vi "save_fp.vi"(7 "Image Type":enum16{"JPEG", "PNG", "BMP"}(ring), 8 "error in":errorcluster, 10 "Image Path":path) -> (0 "error out":errorcluster)   [LabVIEW 2014]
uses:
  <vilib>/Utility/sysdir.llb/System Directory Type.ctl
  type definitions/control camera properties.ctl
panel:
  in  "input cluster 2":T1={"Packet Size"=1500, "Pixel Format"=17825797, "Gain in dB"=1.0, "Exposure Time in µs"=1500, "Stream Bytes per Second"=50000017} caption="Control Camera Properties" {"Stream Bytes per Second" min=1000000 max=124000000 step=100000 format="%.1p"; "Exposure Time in µs" min=21 max=153391689 format="%#.0f"; "Gain in dB" min=0.0 max=26.0 format="%#_2g"; "Pixel Format" items=["Mono 12 Packed"=17563654, "Mono 12"=17825797]}
  in  "input cluster":T2
  out "Image Pixels (U16)":u16[][](graph)
  in  "Image Pixels (U16) 3":u16[][](graph)
  in  "file path":path
  in  "base path":path
  in  "Image Pixels (U16) 2":u16[][](graph)
  # "Bytes"
  # "Trigger"
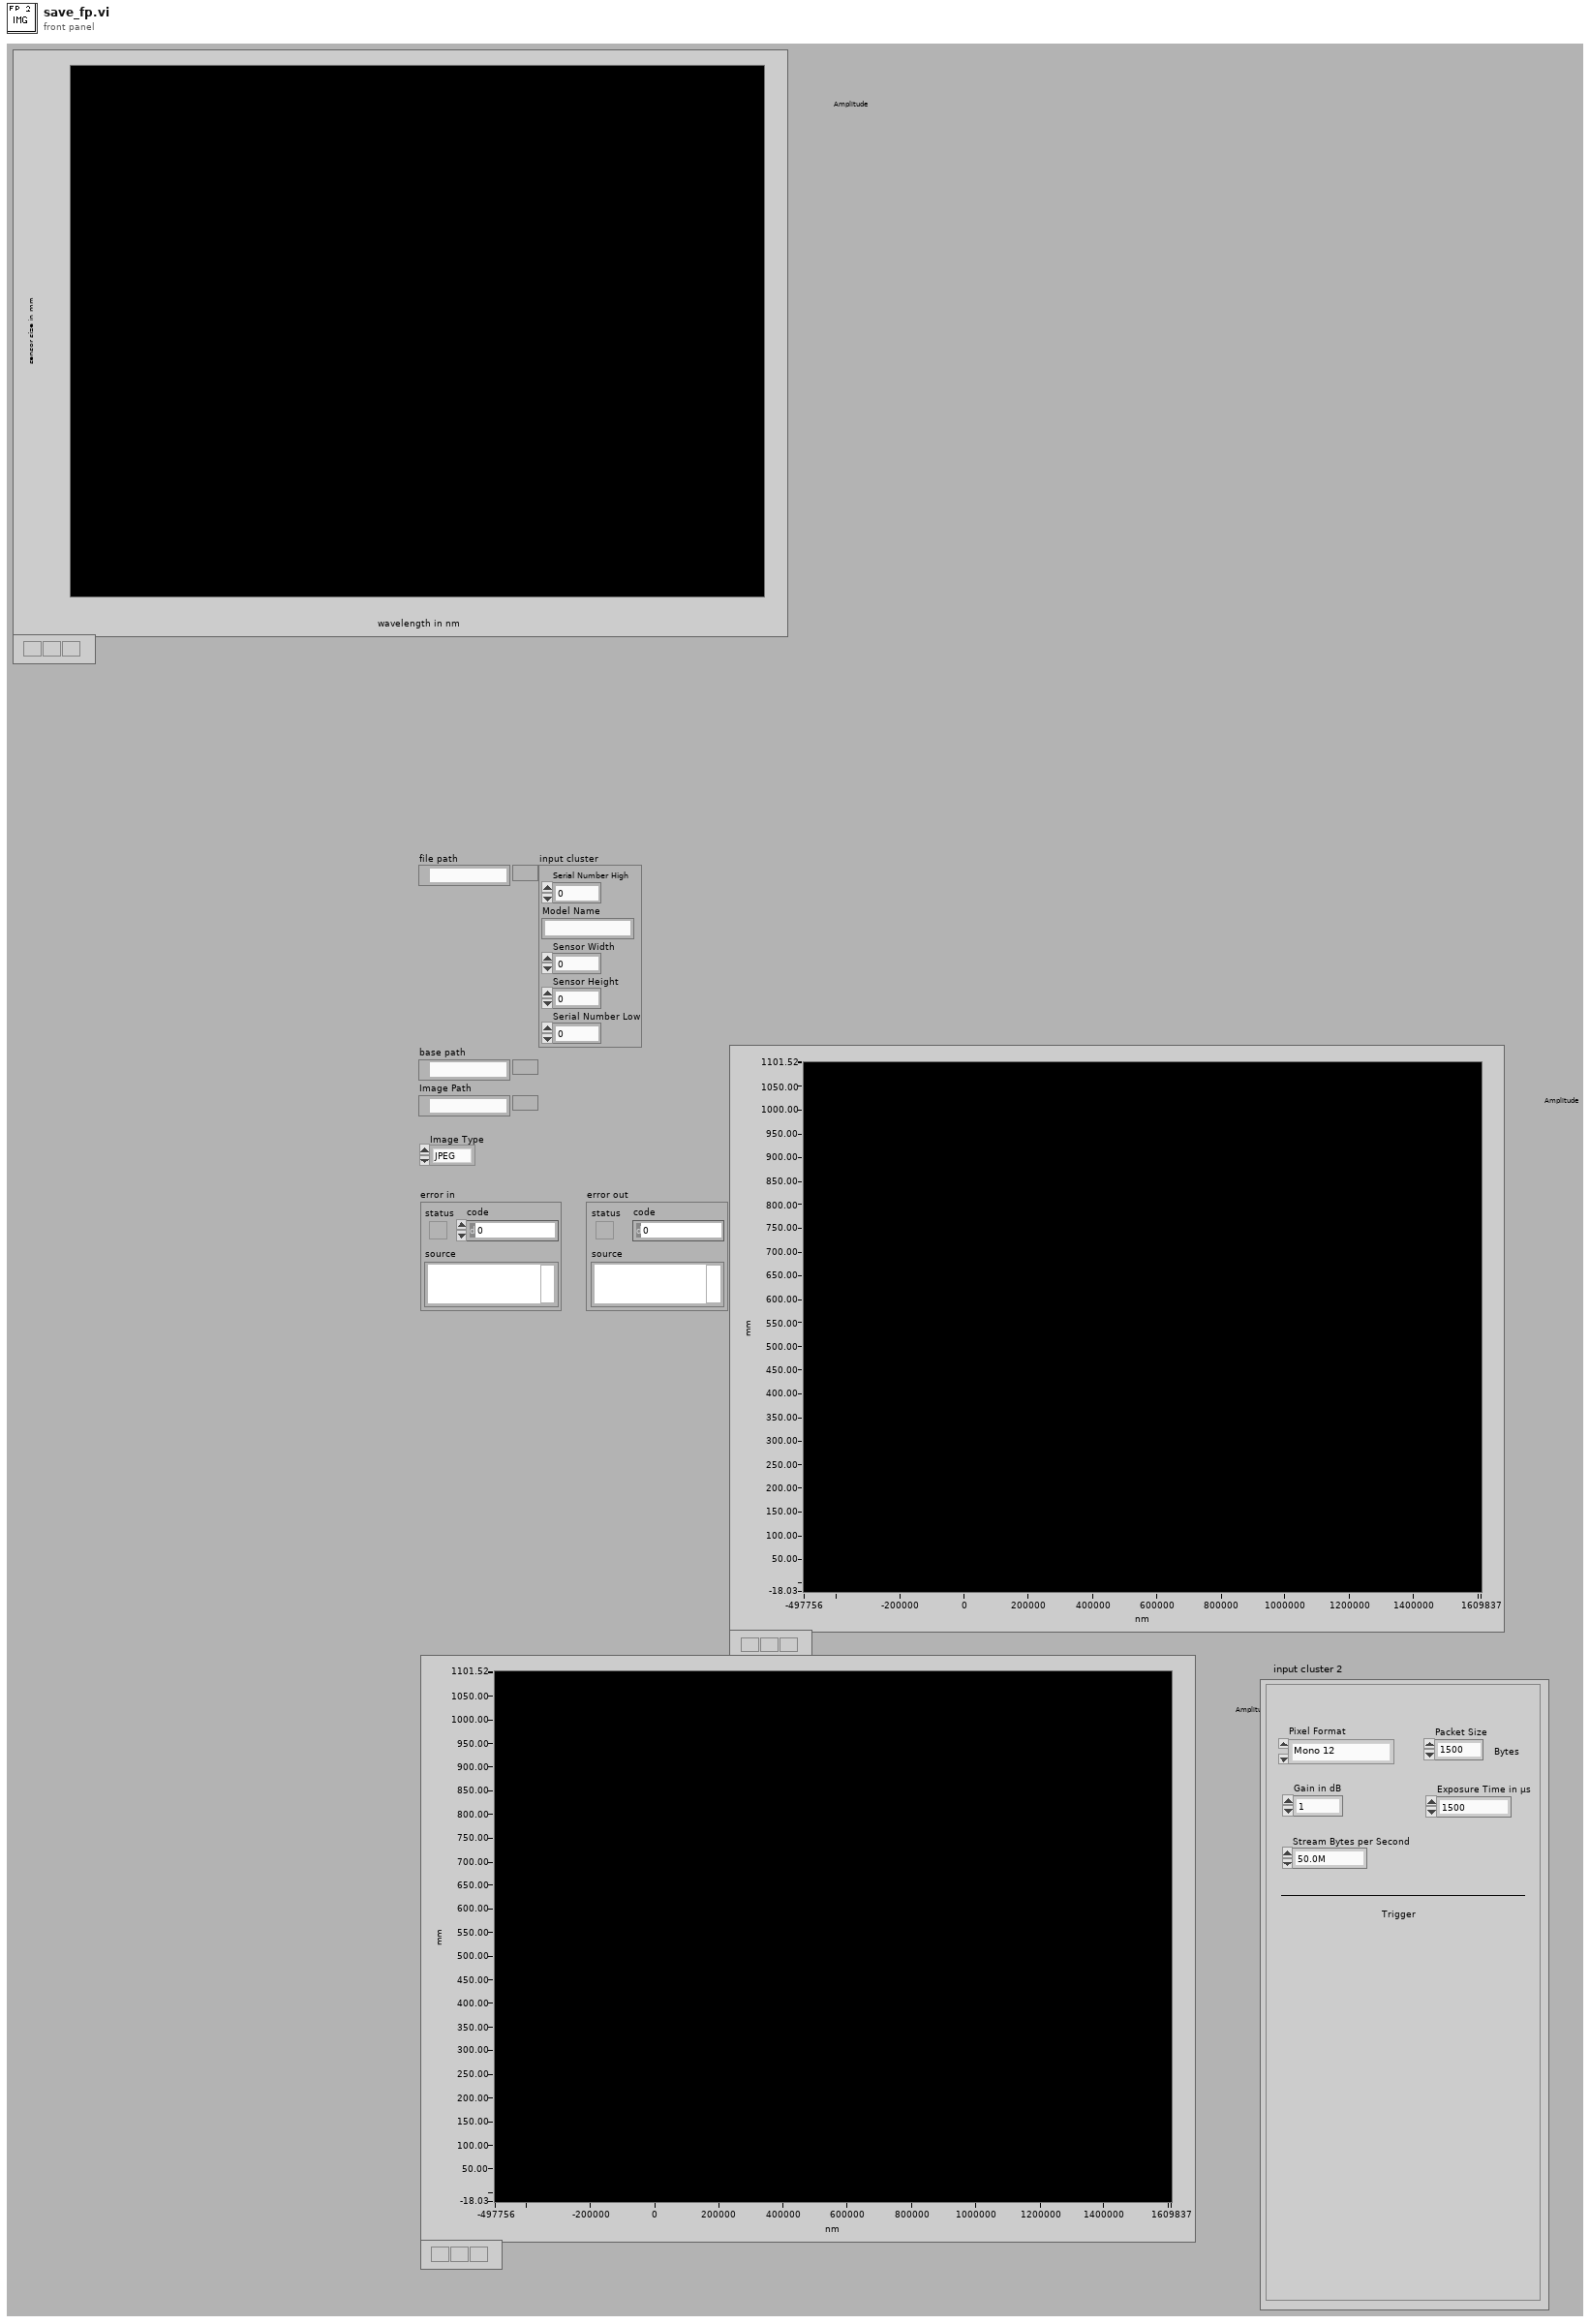
[diagram p1: front panel]
types:
  T1 = typedef "control camera properties.ctl" = cluster{"Packet Size":u32, "Pixel Format":u32, "Gain in dB":dbl, "Exposure Time in µs":u32, "Stream Bytes per Second":u32}
  T2 = cluster{"Serial Number High":u32, "Model Name":string, "Sensor Width":u32, "Sensor Height":u32, "Serial Number Low":u32}
  T3 = enum16{"open", "open or create", "create or replace", "create", "open (read-only)"}
  T4 = typedef "System Directory Type.ctl" = i32
  T5 = enum16{"open", "replace", "create", "open or create", "replace or create", "replace or create with confirmation"}
  T6 = typedef "imagedata.ctl" = cluster{"image type":i32, "image depth":i32, "image":u8[], "mask":u8[], "colors":u32[], "Rectangle":cluster{"left":i16, "top":i16, "right":i16, "bottom":i16}}
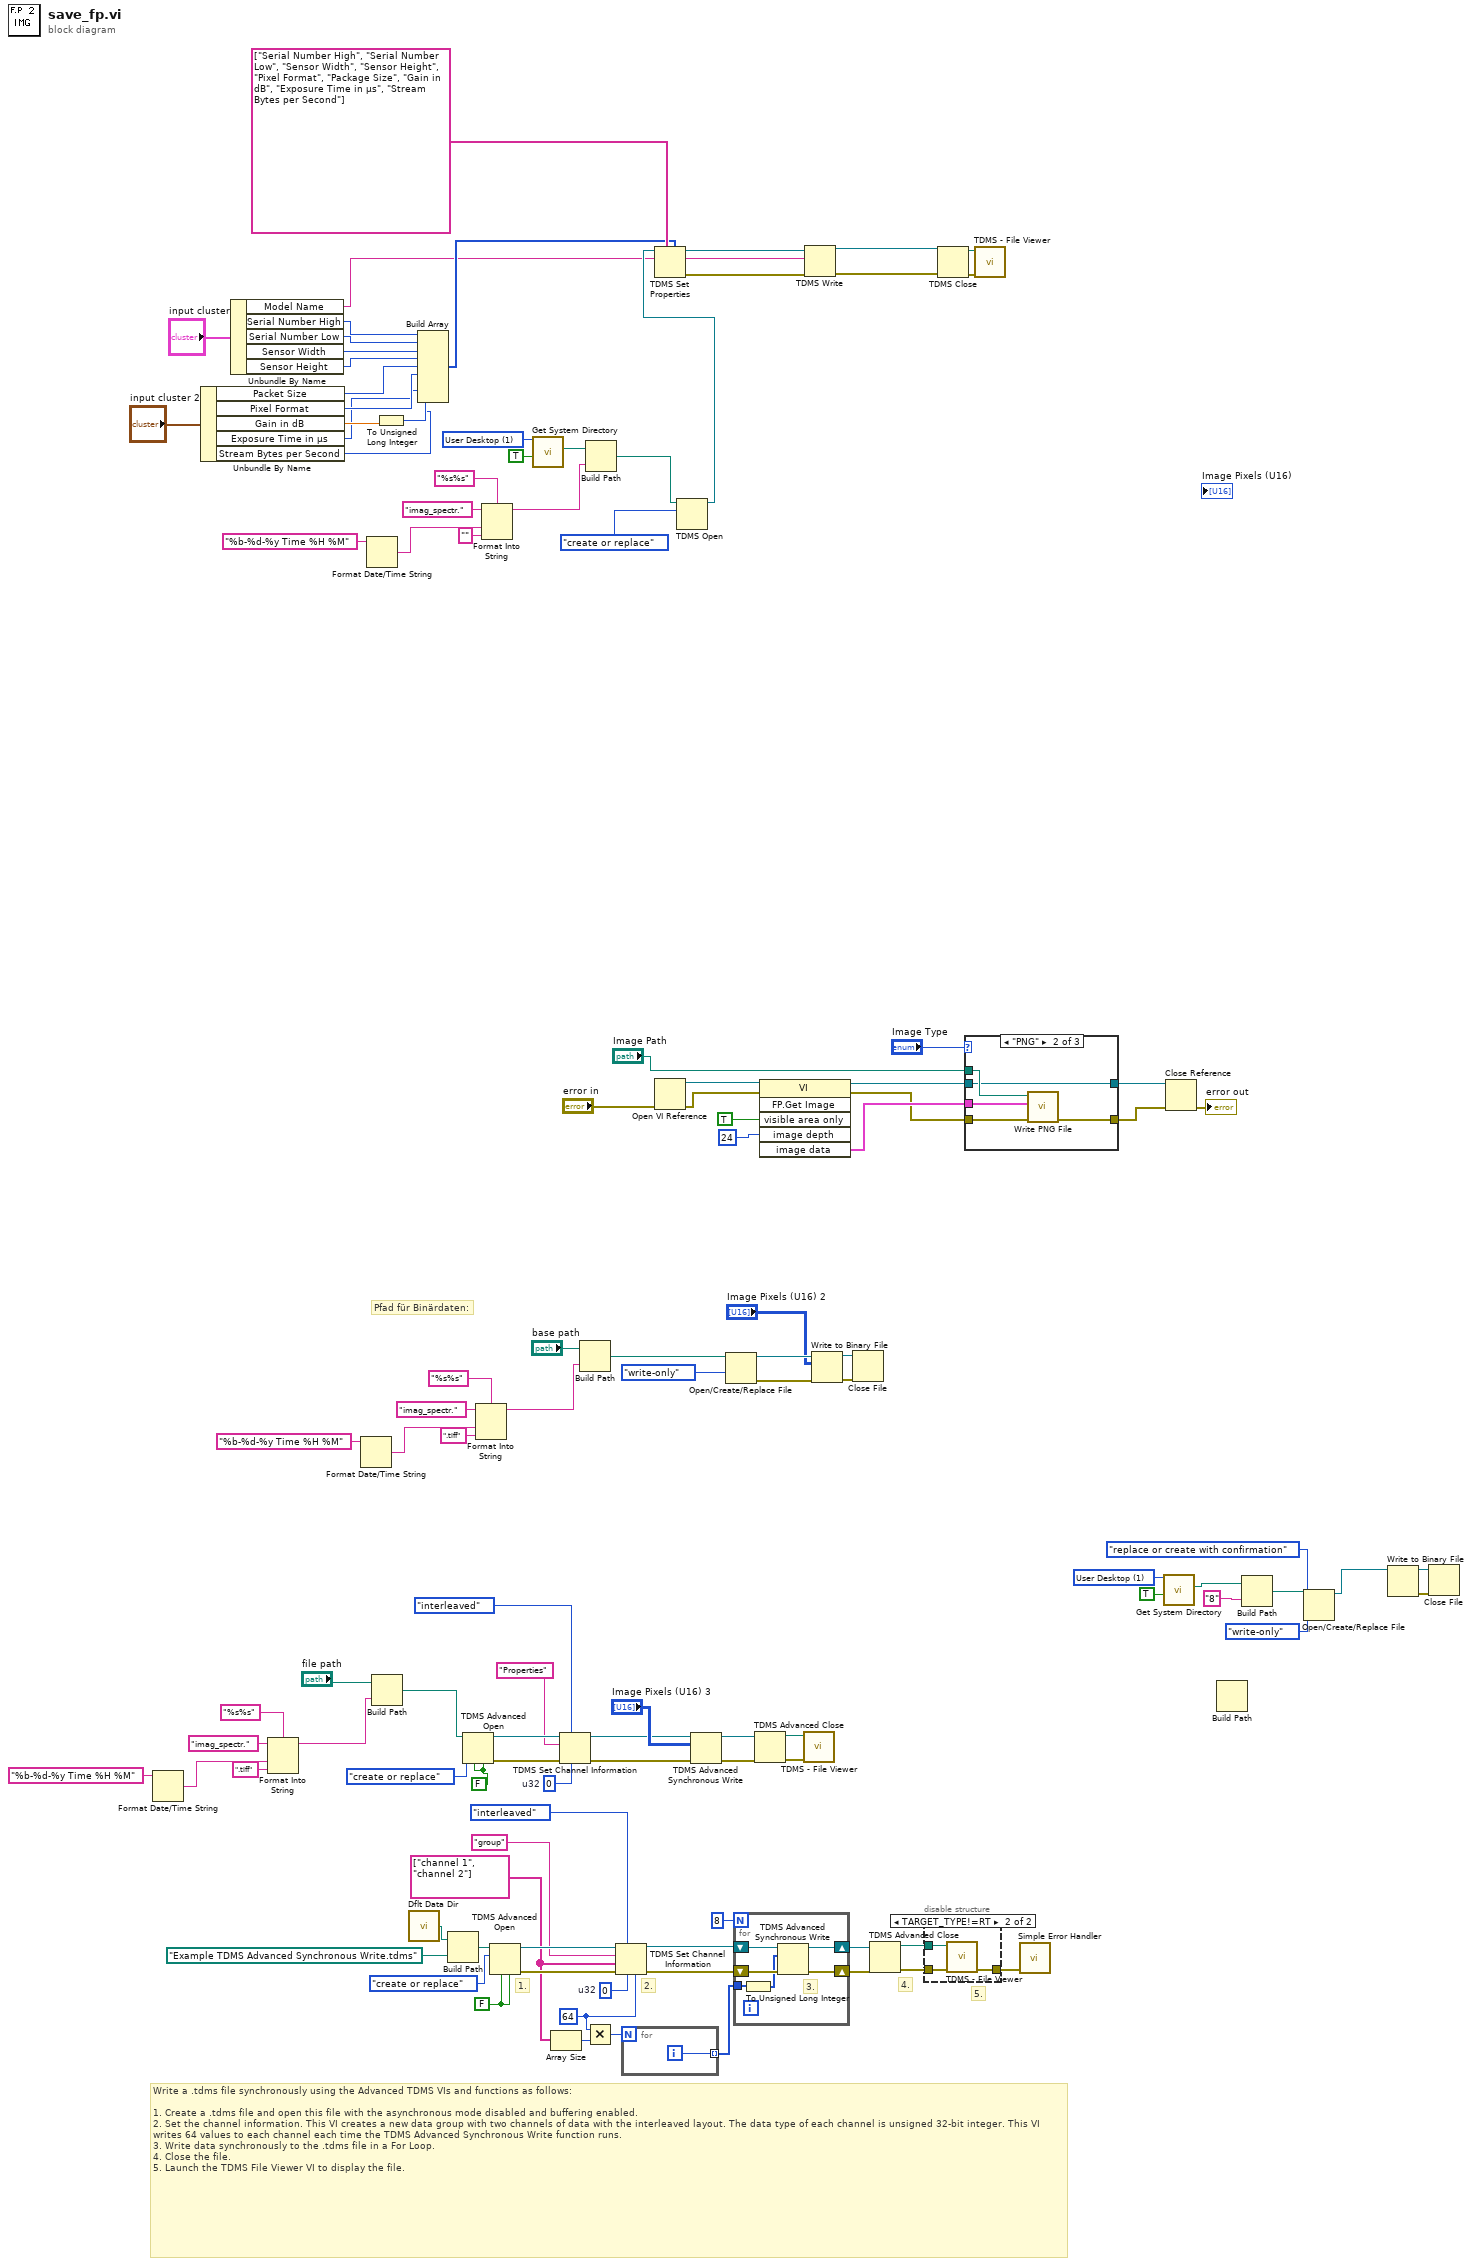
[diagram p0: block diagram]
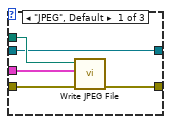
[diagram p3: hidden frame]
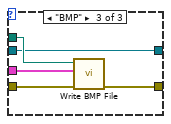
[diagram p4: hidden frame]
diagram:
  w27 = T4 1 items=["User Home"=0, "User Desktop"=1, "User Documents"=2, "User Application Data"=3, "User Preferences"=4, "User Temporary"=5, "Public Documents"=6, "Public Application Data"=7, "Public Preferences"=8, "Public Cache"=13, "System Core Libraries"=9, "System Installed Libraries"=10, "Application Files"=11, "Boot Volume Root"=12] ("system directory type")
  w38 = T4 1 items=["User Home"=0, "User Desktop"=1, "User Documents"=2, "User Application Data"=3, "User Preferences"=4, "User Temporary"=5, "Public Documents"=6, "Public Application Data"=7, "Public Preferences"=8, "Public Cache"=13, "System Core Libraries"=9, "System Installed Libraries"=10, "Application Files"=11, "Boot Volume Root"=12] ("system directory type")
  w56 = u32 0  # u32
  w57 = FALSE
  w76 = FALSE ("enable asynchronous? (T)")
  w66 = u32 64 ("samples per channel")
  w77 = u32 0  # u32
  w67 = string[] ["channel 1", "channel 2"] ("channel name(s)")
  # "Write a .tdms file synchronously using the Advanced TDMS VIs and functions as follows:\n\n1. Create a .tdms file and open this file with the asynchronous mode disabled and buffering enabled.\n2. Set the channel information. This VI creates a new data group with two channels of data with the interleaved layout. The data type of each channel is unsigned 32-bit integer. This VI writes 64 values to each channel each time the TDMS Advanced Synchronous Write function runs.\n3. Write data synchronously to the .tdms file in a For Loop.\n4. Close the file.\n5. Launch the TDMS File Viewer VI to display the file."
  # "5."
  # "1."
  # "4."
  # "2."
  # "Pfad für Binärdaten:"
  n1 = Format Date/Time String(time format string (%c)="%b-%d-%y Time %H %M") -> (date/time string=w60:string)  [unwired: 2 in]
  n2 = Unbundle By Name("input cluster 2") -> ("Packet Size"=w11:u32, "Pixel Format"=w10:u32, "Gain in dB"=w9:dbl, "Exposure Time in µs"=w7:u32, "Stream Bytes per Second"=w6:u32)
  n3 = Unbundle By Name("input cluster") -> ("Model Name"=w4:string, "Serial Number High"=w15:u32, "Serial Number Low"=w14:u32, "Sensor Width"=w13:u32, "Sensor Height"=w12:u32)
  n4 = Format Into String(format string="%s%s", initial string="imag_spectr.", w60, ".tiff" ("input 2")) -> (resulting string=w65:string)  [unwired: 1 in, 1 out]
  n5 = Format Date/Time String(time format string (%c)="%b-%d-%y Time %H %M") -> (date/time string=w103:string)  [unwired: 2 in]
  n6 = Format Date/Time String(time format string (%c)="%b-%d-%y Time %H %M") -> (date/time string=w21:string)  [unwired: 2 in]
  n7 = Build Path(base path="file path", name or relative path=w65) -> (appended path=w58:path)
  n8 = To Unsigned Long Integer(number=w9) -> (unsigned 32bit integer=w8:u32)
  n9 = call <vilib>:"Dflt Data Dir.vi"() -> ("App:Default Data Directory"=w84:path)
  n10 = Build Array(w15, w14, w13, w12, w11, w10, w8, w7, w6) -> (w5:u32[])
  n11 = Build Path(base path=w84, name or relative path=path "Example TDMS Advanced Synchronous Write.tdms") -> (appended path=w88:path)
  n12 = TDMS Advanced Open(4:w57, 6:w57, 10:T3."create or replace" ("operation (0:open)"), 11:w58) -> (0:w55:errorcluster, 3:w54:refnum<k34>)  [unwired: 1 in, 1 out]
  n13 = Format Into String(format string="%s%s", initial string="imag_spectr.", w103, ".tiff" ("input 2")) -> (resulting string=w89:string)  [unwired: 1 in, 1 out]
  n14 = Format Into String(format string="%s%s", initial string="imag_spectr.", w21, "" ("input 2")) -> (resulting string=w25:string)  [unwired: 1 in, 1 out]
  n15 = TDMS Advanced Open(4:w76, 6:w76, 10:T3."create or replace" ("operation (0:open)"), 11:w88) -> (0:w86:errorcluster, 3:w85:refnum<k34>)  [unwired: 1 in, 1 out]
  n16 = call <vilib>:"Get System Directory.vi"("create directory if not found? (F)"=TRUE, "system directory type"=w27) -> ("system directory"=w20:path)  [unwired: 9 in]
  n17 = Array Size(array=w67) -> (size(s)=w69:i32)
  n18 = TDMS Set Channel Information(6:w56, 7:enum16{"non-interleaved", "interleaved"}."interleaved" ("data layout (0:non-interleaved)"), 8:w55, 10:"Properties" ("group name (Untitled)"), 11:w54) -> (0:w49:errorcluster, 3:w50:refnum<k34>)  [unwired: 2 in]
  n19 = Build Path(base path="base path", name or relative path=w89) -> (appended path=w96:path)
  n20 = Multiply(x=w66, y=w69) -> (x*y=w68:u32)
  n21 = Build Path(base path=w20, name or relative path=w25) -> (appended path=w2:path)
  n22 = TDMS Set Channel Information(4:w66, 6:w77, 7:enum16{"non-interleaved", "interleaved"}."interleaved" ("data layout (0:non-interleaved)"), 8:w86, 9:w67, 10:"group" ("group name (Untitled)"), 11:w85) -> (0:w75:errorcluster, 3:w74:refnum<k34>)
  n23 = for {
    N: w68 -> [_]
    tunnel: [w117] -> w80 mode=indexing
    i -> [w117]
  }
  n24 = Open VI Reference(error in (no error)="error in") -> (vi reference=w114:refnum<vi>, error out=w113:errorcluster)  [unwired: 2 in, 3 out]
  n25 = TDMS Open(10:T3."create or replace" ("operation (0:open)"), 11:w2) -> (3:w18:refnum<k34>)  [unwired: 5 in, 1 out]
  n26 = TDMS Set Properties(5:w5, 7:string[] ["Serial Number High", "Serial Number Low", "Sensor Width", "Sensor Height", "Pixel Format", "Package Size", "Gain in dB", "Exposure Time in µs", "Stream Bytes per Second"] ("property names"), 10:w4, 11:w18) -> (0:w17:errorcluster, 2:w3:string, 3:w16:refnum<k34>)  [unwired: 2 in, 1 out]
  n27 = TDMS Advanced Synchronous Write(8:w49, 10:"Image Pixels (U16) 3", 11:w50) -> (0:w47:errorcluster, 3:w48:refnum<k34>)
  n28 = Open/Create/Replace File(file path (use dialog)=w96, access (0:read/write)=enum16{"read/write", "read-only", "write-only"}."write-only") -> (refnum out=w95:refnum<file>, error out=w92:errorcluster)  [unwired: 4 in, 1 out]
  n29 = for {
    N: 8 -> [_]
    shift-right: [w120] -> w78
    shift-left: w74 -> [w122]
    shift-right: [w121] -> w79
    shift-left: w75 -> [w123]
    tunnel: w80 -> [w119]
    # "3."
    n30 = To Unsigned Long Integer(number=w119) -> (unsigned 32bit integer=w118:u32[])
    n31 = TDMS Advanced Synchronous Write(8:w123, 10:w118, 11:w122) -> (0:w121:errorcluster, 3:w120:refnum<k34>)
  }
  n32 = TDMS Advanced Close(8:w47, 11:w48) -> (0:w46:errorcluster, 3:w45:path)  [unwired: 2 in]
  n33 = invoke class="VI" method="FP.Get Image"(reference=w114, error in=w113, "visible area only"=TRUE ("Visible Area Only"), "image depth"=24 ("Image Depth")) -> (reference out=w107:refnum<vi>, error out=w110:errorcluster, "image data"=w111:T6)  [unwired: 2 in, 3 out]
  n34 = call <vilib>:"TDMS - File Viewer.vi"("error in (no error)"=w46, "file path"=w45) -> ()  [unwired: 6 out]
  n35 = TDMS Write(0:w16, 5:w3, 11:w17) -> (4:w30:refnum<k34>, 15:w31:errorcluster)  [unwired: 3 in, 2 out]
  n36 = Write to Binary File(file (use dialog)=w95, data="Image Pixels (U16) 2", error in=w92) -> (refnum out=w94:refnum<file>, error out=w97:errorcluster)  [unwired: 3 in, 1 out]
  n37 = Close File(refnum=w94, error in=w97) -> ()  [unwired: 2 out]
  n38 = TDMS Advanced Close(8:w79, 11:w78) -> (0:w71:errorcluster, 3:w72:path)  [unwired: 2 in]
  n39 = disable-structure shown="TARGET_TYPE!=RT" {
    disable-tunnel: w71 -> [w124 w127]
    disable-tunnel: w72 -> [_ w126]
    disable-tunnel: [w124 w125] -> w70
    frame condition #0 {
    }
    frame condition #1 (active) {
      n40 = call <vilib>:"TDMS - File Viewer.vi"("error in (no error)"=w127, "file path"=w126) -> ("error out"=w125:errorcluster)  [unwired: 5 out]
    }
  }
  n41 = TDMS Close(8:w31, 11:w30) -> (0:w32:errorcluster, 3:w29:path)
  n42 = case shown="\"PNG\"" "Image Type" {
    tunnel: w111 -> [w131 w137 w141]
    tunnel: w110 -> [w132 w136 w142]
    tunnel: "Image Path" -> [w130 w135 w140]
    tunnel: [w128 w134 w139] -> w108
    tunnel: w107 -> [w129 w133 w138]
    tunnel: [w129 w133 w138] -> w106
    frame "JPEG", Default {
      n43 = call <vilib>:"Write JPEG File.vi"("error in (no error)"=w132, "image data"=w131, "path to JPEG file"=w130) -> ("error out"=w128:errorcluster)  [unwired: 8 out]
    }
    frame "PNG" {
      n44 = call <vilib>:"Write PNG File.vi"("error in (no error)"=w136, "image data"=w137, "path to PNG file"=w135) -> ("error out"=w134:errorcluster)  [unwired: 8 out]
    }
    frame "BMP" {
      n45 = call <vilib>:"Write BMP File.vi"("error in (no error)"=w142, "image data"=w141, "path to BMP file"=w140) -> ("error out"=w139:errorcluster)  [unwired: 8 out]
    }
  }
  n46 = call <vilib>:"TDMS - File Viewer.vi"("error in (no error)"=w32, "file path"=w29) -> ()  [unwired: 4 in, 2 out]
  n47 = call <vilib>:"Simple Error Handler.vi"("error in (no error)"=w70) -> ()  [unwired: 4 in, 5 out]
  n48 = call <vilib>:"Get System Directory.vi"("create directory if not found? (F)"=TRUE, "system directory type"=w38) -> ("system directory"=w35:path)  [unwired: 9 in]
  n49 = Close Reference(reference=w106, error in (no error)=w108) -> (error out=→"error out":errorcluster)
  n50 = Build Path() -> ()  [unwired: 2 in, 1 out]
  n51 = Build Path(base path=w35, name or relative path="8") -> (appended path=w43:path)
  n52 = Open/Create/Replace File(file path (use dialog)=w43, operation (0:open)=T5."replace or create with confirmation", access (0:read/write)=enum16{"read/write", "read-only", "write-only"}."write-only") -> (refnum out=w40:refnum<file>)  [unwired: 3 in, 2 out]
  n53 = Write to Binary File(file (use dialog)=w40) -> (refnum out=w36:refnum<file>, error out=w37:errorcluster)  [unwired: 5 in, 1 out]
  n54 = Close File(refnum=w36, error in=w37) -> ()  [unwired: 2 out]
